vi "PDF Einheiten in Tabellenheader.vi"(7 "TestKonfig":T1 {"TestKonfig Interferent"."Gasflasche MFC3" items=["----"=10000, "IAG NH3 3000"=0, "IAG NH3 200"=1, "IAG NH3 2000"=2, "IAG MG"=3, "IAG O2"=4]; "TestKonfig Interferent"."Gasflasche MFC2" items=["----"=10000, "IAG NH3 3000"=0, "IAG NH3 200"=1, "IAG NH3 2000"=2, "IAG MG"=3, "IAG O2"=4]; "TestKonfig Interferent"."Eingangs Konzentration MFC1" min=0.0; "TestKonfig Interferent"."Ausgangs Konzentration MFC1" min=0.0; "TestKonfig Interferent"."MFC2" items=["MFC 2", "MFC 3", "MFC 4", "MFC 5"]; "TestKonfig Interferent"."MFC3" items=["MFC 2", "MFC 3", "MFC 4", "MFC 5"]; "TestKonfig Interferent"."Ausgangs Konzentration MFC3" min=0.0; "TestKonfig Interferent"."Eingangs Konzentration MFC3" min=0.0; "TestKonfig Interferent"."Ausgangs Konzentration MFC2" min=0.0; "TestKonfig Interferent"."Eingangs Konzentration MFC2" min=0.0; "TestKonfig H2O"."HovaCAL Temperature" format="%.2f"; "TestKonfig H2O"."HovaCAL Flow Input Cluster"."HovaCAL Flow Input Cluster" format="%.2f"; "TestKonfig H2O"."Eingangs Konzentration:" min=0.0; "TestKonfig H2O"."zusätzliche Zeitdauer Erster Punkt" min=30 step=1 format="%#_5g"; "TestKonfig H2O"."Zeitdauer Stufen" format="%#_5g"; "TestKonfig H2O"."Max Fehler" format="%#_5g"; "TestKonfig H2O"."Anzahl Stufen" format="%#_5g"; "TestKonfig H2O"."Modus" items=["Messen", "CG zu Entnahmestelle"]}, 8 "error in (no error)":errorcluster caption="Fehler (Eingang, kein Fehler)", 9 "Kontroll Interferent LIN Ausgabetabelle":refnum<vi>, 10 "Referenz Interferent LIN Ausgabetabelle":refnum<vi>, 11 "Tabelle (Eingang)":refnum<vi>) -> (0 "Fehler (Ausgang)":errorcluster)   [LabVIEW 2020, in "EPA 1065.lvlib" / "HovaCAL Interference verificaton.lvlib"]
uses:
  HovaCAL Interference verificaton.lvlib
  TestKonfig.ctl
  TestKonfig H2O.ctl
  Modus.ctl
  Linearisierung V2/SpanEinstellungen/Einheit.ctl
  Linearisierung V2/Gasteiler/Stufen Tabelle.ctl
  Linearisierung V2/Gasteiler/HovaCAL_Interface/Controls/Flow Einstellung.ctl
  Linearisierung V2/Gasteiler/HovaCAL_Interface/Controls/Temp Sollwerte Anzeige.ctl
  TestKonfig Interferents.ctl
  MFCAuswahl.ctl
  Seiten/System Einstellungen V2/Gasflasche Auswahl.ctl
  Linearisierung V2/Linearisierung v2.lvlib
  Linearisierung V2/SpanEinstellungen/SpanEinstellungen.lvlib
  Linearisierung V2/Gasteiler/Gasteiler.lvlib
  Linearisierung V2/Gasteiler/HovaCAL_Interface/Controls/Controls.lvlib
  Seiten/System Einstellungen V2/System Einstellungen V2.lvlib
panel:
  # "sec"
  # "%"
  # "sec"
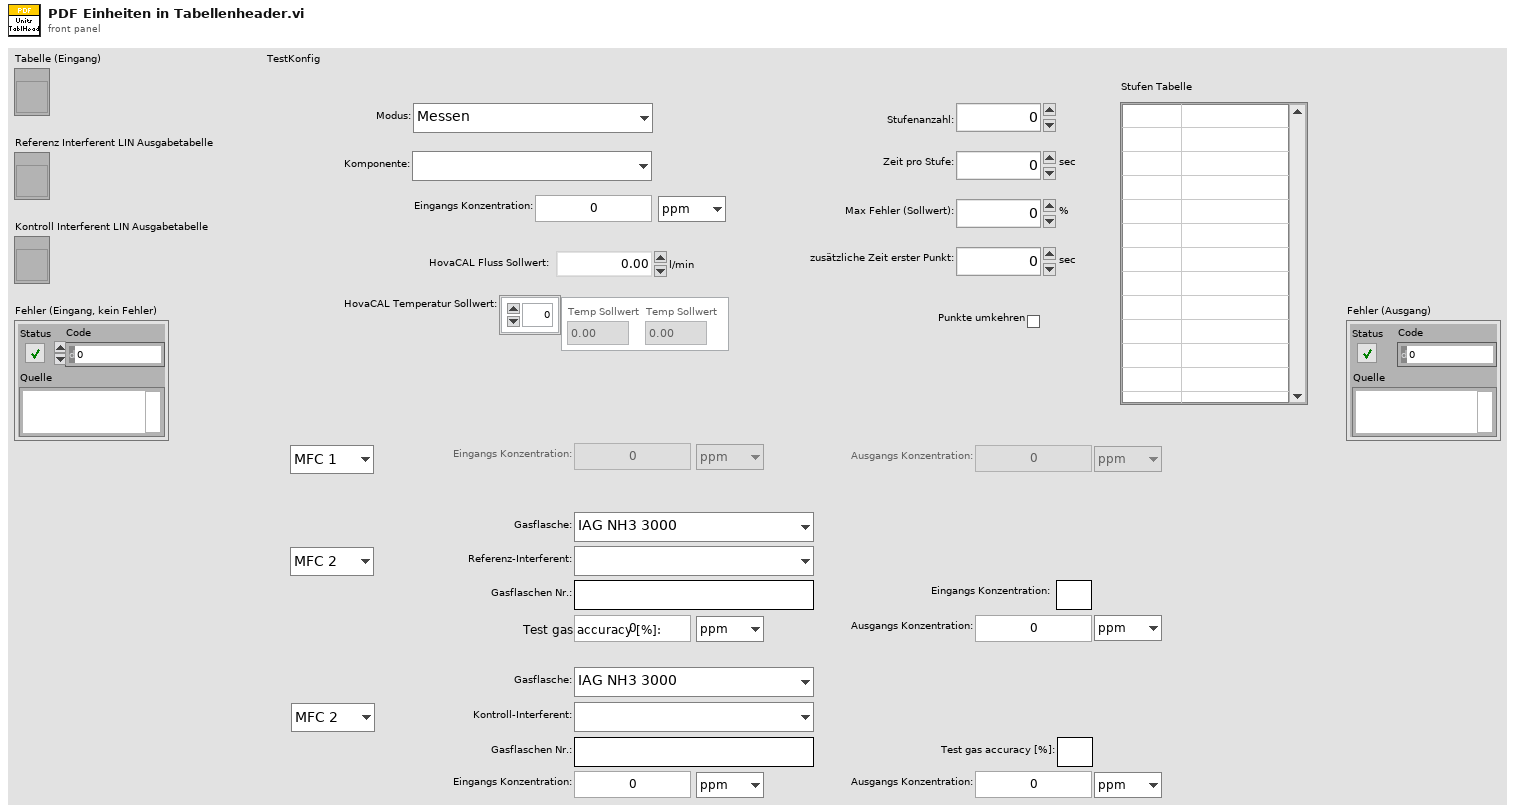
[diagram p1: front panel]
types:
  T1 = typedef "EPA 1065.lvlib/HovaCAL Interference verificaton.lvlib/TestKonfig.ctl" = cluster{"TestKonfig H2O":T2, "TestKonfig Interferent":T8}
  T2 = typedef "EPA 1065.lvlib/HovaCAL Interference verificaton.lvlib/TestKonfig H2O.ctl" = cluster{"Modus":T3, "Komponente:":u16, "Eingangs Konzentration:":dbl, "Einheit":T4, "Anzahl Stufen":sgl, "Zeitdauer Stufen":sgl, "Max Fehler":sgl, "zusätzliche Zeitdauer Erster Punkt":sgl, "Punkte umkehren":bool, "Stufen Tabelle":T5, "HovaCAL Flow Input Cluster":T6, "HovaCAL Temperature":T7}
  T3 = typedef "EPA 1065.lvlib/HovaCAL Interference verificaton.lvlib/Modus.ctl" = u16
  T4 = typedef "Linearisierung v2.lvlib/SpanEinstellungen.lvlib/Einheit.ctl" = enum16{"ppm", "%"}
  T5 = typedef "Linearisierung v2.lvlib/Gasteiler.lvlib/Stufen Tabelle.ctl" = string[][]
  T6 = typedef "Linearisierung v2.lvlib/Gasteiler.lvlib/HovaCAL_Interface.lvlib/Controls.lvlib/Flow Einstellung.ctl" = cluster{"HovaCAL Flow Input Cluster":dbl}
  T7 = typedef "Linearisierung v2.lvlib/Gasteiler.lvlib/HovaCAL_Interface.lvlib/Controls.lvlib/Temp Sollwerte Anzeige.ctl" = dbl[]
  T8 = typedef "EPA 1065.lvlib/HovaCAL Interference verificaton.lvlib/TestKonfig Interferents.ctl" = cluster{"MFC1":enum16{"MFC 1"}, "Eingangs Konzentration MFC1":dbl, "Einheit MFC1 Eingang":T4, "Ausgangs Konzentration MFC1":dbl, "Einheit MFC1 Ausgang":T4, "MFC2":T9, "Referenz-Interferent:":u16, "Gasflaschen Nr MFC2":string, "Accuracy MFC2":string, "Eingangs Konzentration MFC2":dbl, "Einheit MFC2 Eingang":T4, "Ausgangs Konzentration MFC2":dbl, "Einheit MFC2 Ausgang":T4, "MFC3":T9, "Kontroll-Interferent:":u16, "Gasflaschen Nr MFC3":string, "Accuracy MFC3":string, "Eingangs Konzentration MFC3":dbl, "Einheit MFC3 Eingang":T4, "Ausgangs Konzentration MFC3":dbl, "Einheit MFC3 Ausgang":T4, "Gasflasche MFC2":T10, "Gasflasche MFC3":T10}
  T9 = typedef "EPA 1065.lvlib/HovaCAL Interference verificaton.lvlib/MFCAuswahl.ctl" = u16
  T10 = typedef "System Einstellungen V2.lvlib/Gasflasche Auswahl.ctl" = u16
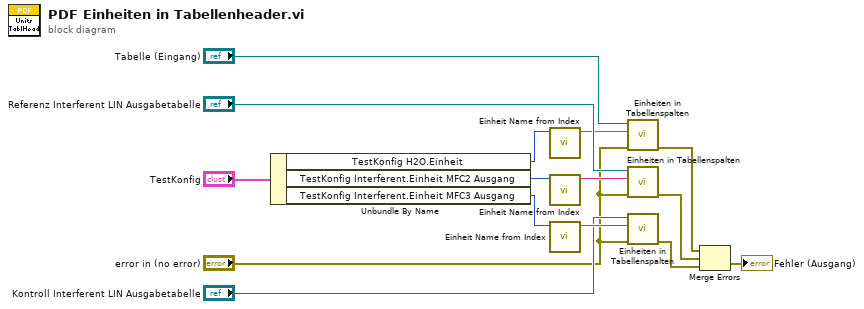
[diagram p0: block diagram]
diagram:
  n1 = Unbundle By Name("TestKonfig") -> ("TestKonfig H2O.Einheit"=w8:T4, "TestKonfig Interferent.Einheit MFC2 Ausgang"=w12:T4, "TestKonfig Interferent.Einheit MFC3 Ausgang"=w14:T4)
  n2 = call "Einheit Name from Index.vi"("EinheitIndex"=w8) -> ("EinheitName"=w9:string)  [unwired: 10 in]
  n3 = call "Einheit Name from Index.vi"("EinheitIndex"=w12) -> ("EinheitName"=w13:string)  [unwired: 10 in]
  n4 = call "Einheit Name from Index.vi"("EinheitIndex"=w14) -> ("EinheitName"=w15:string)  [unwired: 10 in]
  n5 = call "Einheiten in Tabellenspalten.vi"("error in (no error)"="error in (no error)", "Einheit"=w9, "Tabelle (Eingang)"="Tabelle (Eingang)") -> ("error out"=w6:errorcluster)  [unwired: 6 in, 2 out]
  n6 = call "Einheiten in Tabellenspalten.vi"("error in (no error)"="error in (no error)", "Einheit"=w13, "Tabelle (Eingang)"="Referenz Interferent LIN Ausgabetabelle") -> ("error out"=w2:errorcluster)  [unwired: 6 in, 2 out]
  n7 = call "Einheiten in Tabellenspalten.vi"("error in (no error)"="error in (no error)", "Einheit"=w15, "Tabelle (Eingang)"="Kontroll Interferent LIN Ausgabetabelle") -> ("error out"=w1:errorcluster)  [unwired: 6 in, 2 out]
  n8 = Merge Errors(w6, w2, w1) -> (→"Fehler (Ausgang)":errorcluster)
